vi "Acquire.vi"(3 "Correction and Conversion":dbl[](array[numeric]), 5 "Timing":T9={"Resolution (ms)"=0.0, "index"=0, "Duty cycle array size"=0, "Pre-scan rest (ms)"=2000}, 7 "Averaging and Conversion":T2, 9 "Method Output":T1, 11 "Data In":dbl[][](array[numeric]), 13 "Average In":dbl[][](array[numeric]), 16 "Calibration?":bool, 19 "Arduino In":cluster{"error in":errorcluster, "LINX  in":T3}) -> (2 "Stop condition":bool, 6 "Acquisition":T10, 10 "Data Out":dbl[][](array[numeric]), 12 "Average Out":dbl[][](array[numeric]), 14 "Arduino Out":cluster{"error out":errorcluster, "LINX out":T3})   [LabVIEW 2022 SP3]
uses:
  <vilib>/MakerHub/LINX/Private/Type Defs/LINX Ref.ctl
  <vilib>/MakerHub/LINX/Private/Type Defs/Platform.ctl
  <vilib>/MakerHub/LINX/Private/Type Defs/Interface.ctl
  <vilib>/MakerHub/LINX/Private/Device/Type Defs/LINX Device Config.ctl
  <vilib>/MakerHub/LINX/Private/Device/Type Defs/TCP Config.ctl
  <vilib>/MakerHub/LINX/Private/Device/Type Defs/Channels.ctl
  <vilib>/MakerHub/LINX/Public/Peripherals/PWM/PWM Set Duty Cycle 1 Chan.vi
  <vilib>/MakerHub/LINX/Public/Peripherals/Analog/Analog Read 1 Chan.vi
  <vilib>/Analysis/baseanly.llb/Mean (DBL).vi
  <vilib>/MakerHub/LINX/Public/Peripherals/Analog/Analog Read N Chans.vi
  <vilib>/MakerHub/LINX/Private/Local IO/LinxAnalogRead.vi
  <vilib>/MakerHub/LINX/Public/Utilities/Check Channel.vi
  <vilib>/MakerHub/LINX/Public/Peripherals/PWM/PWM Set Duty Cycle N Chans.vi
  <vilib>/MakerHub/LINX/Private/Utilties/Generate Error.vi
  <vilib>/MakerHub/LINX/LMH-LINX.lvlib
  <vilib>/Analysis/NI_AALBase.lvlib
  <vilib>/MakerHub/LINX/Private/Device/Device.lvlib
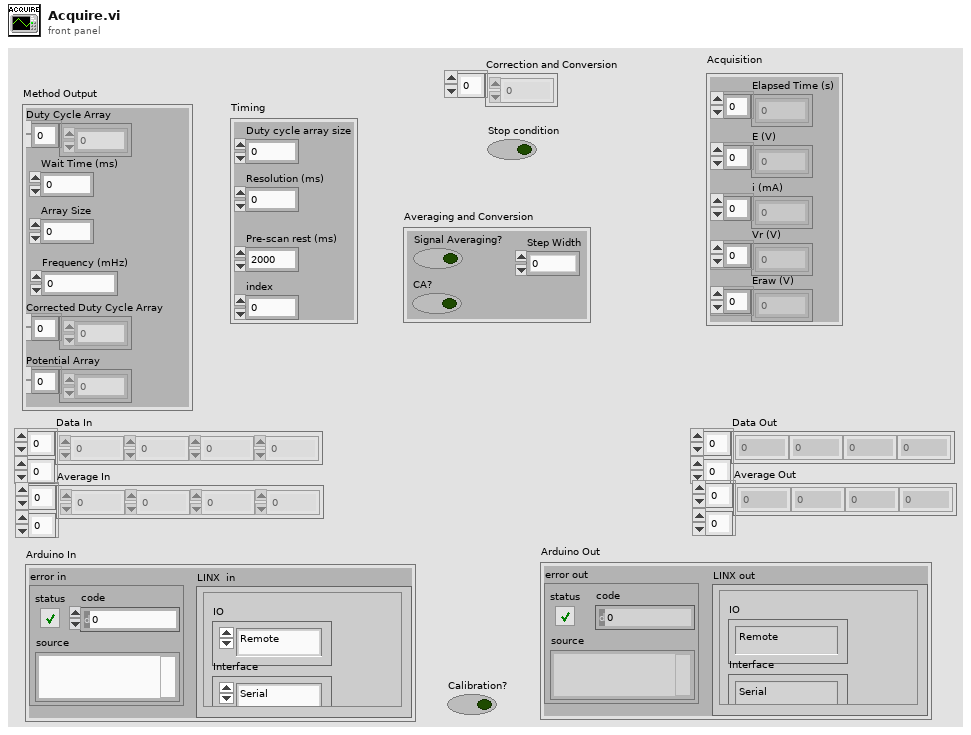
[diagram p1: front panel]
types:
  T1 = cluster{"Duty Cycle Array":dbl[], "Wait Time (ms)":dbl, "Array Size":i32, "Frequency (mHz)":dbl, "Corrected Duty Cycle Array":dbl[], "Potential Array":dbl[]}
  T2 = cluster{"Signal Averaging?":bool, "CA?":bool, "Step Width":dbl}
  T3 = typedef "LMH-LINX.lvlib/LINX Ref.ctl" = cluster{"IO":T4, "Interface":T5, "LINX Device Config":T6}
  T4 = typedef "LMH-LINX.lvlib/Platform.ctl" = enum16{"Remote", "Local"}
  T5 = typedef "LMH-LINX.lvlib/Interface.ctl" = enum16{"Serial", "TCP"}
  T6 = typedef "LMH-LINX.lvlib/Device.lvlib/LINX Device Config.ctl" = cluster{"Interface":T5, "COM Port":refnum<visa-resource-name>, "TCP Configuration":T7, "Device Family":u8, "Device ID":u8, "Device Name":string, "TCP Ref":refnum<k5>, "Channels":T8}
  T7 = typedef "LMH-LINX.lvlib/Device.lvlib/TCP Config.ctl" = cluster{"IP Address":string, "Port":u16}
  T8 = typedef "LMH-LINX.lvlib/Channels.ctl" = cluster{"DI":u8[], "DO":u8[], "AI":u8[], "AO":u8[], "PWM":u8[], "QE":u8[], "UART":u8[], "I2C 2":u8[], "SPI":u8[], "CAN":u8[], "Servo":u8[], "AI Ref (V)":dbl, "AI Resolution (Bits)":u8, "AO Ref (V)":dbl, "AO Resolution (Bits)":u8}
  T9 = cluster{"Resolution (ms)":dbl, "index":i32, "Duty cycle array size":i32, "Pre-scan rest (ms)":u32}
  T10 = cluster{"Elapsed Time (s)":dbl[], "E (V)":dbl[], "i (mA)":dbl[], "Vr (V)":dbl[], "Eraw (V)":dbl[]}
  T11 = cluster{"Error Out":errorcluster, "LINX Resource":T3}
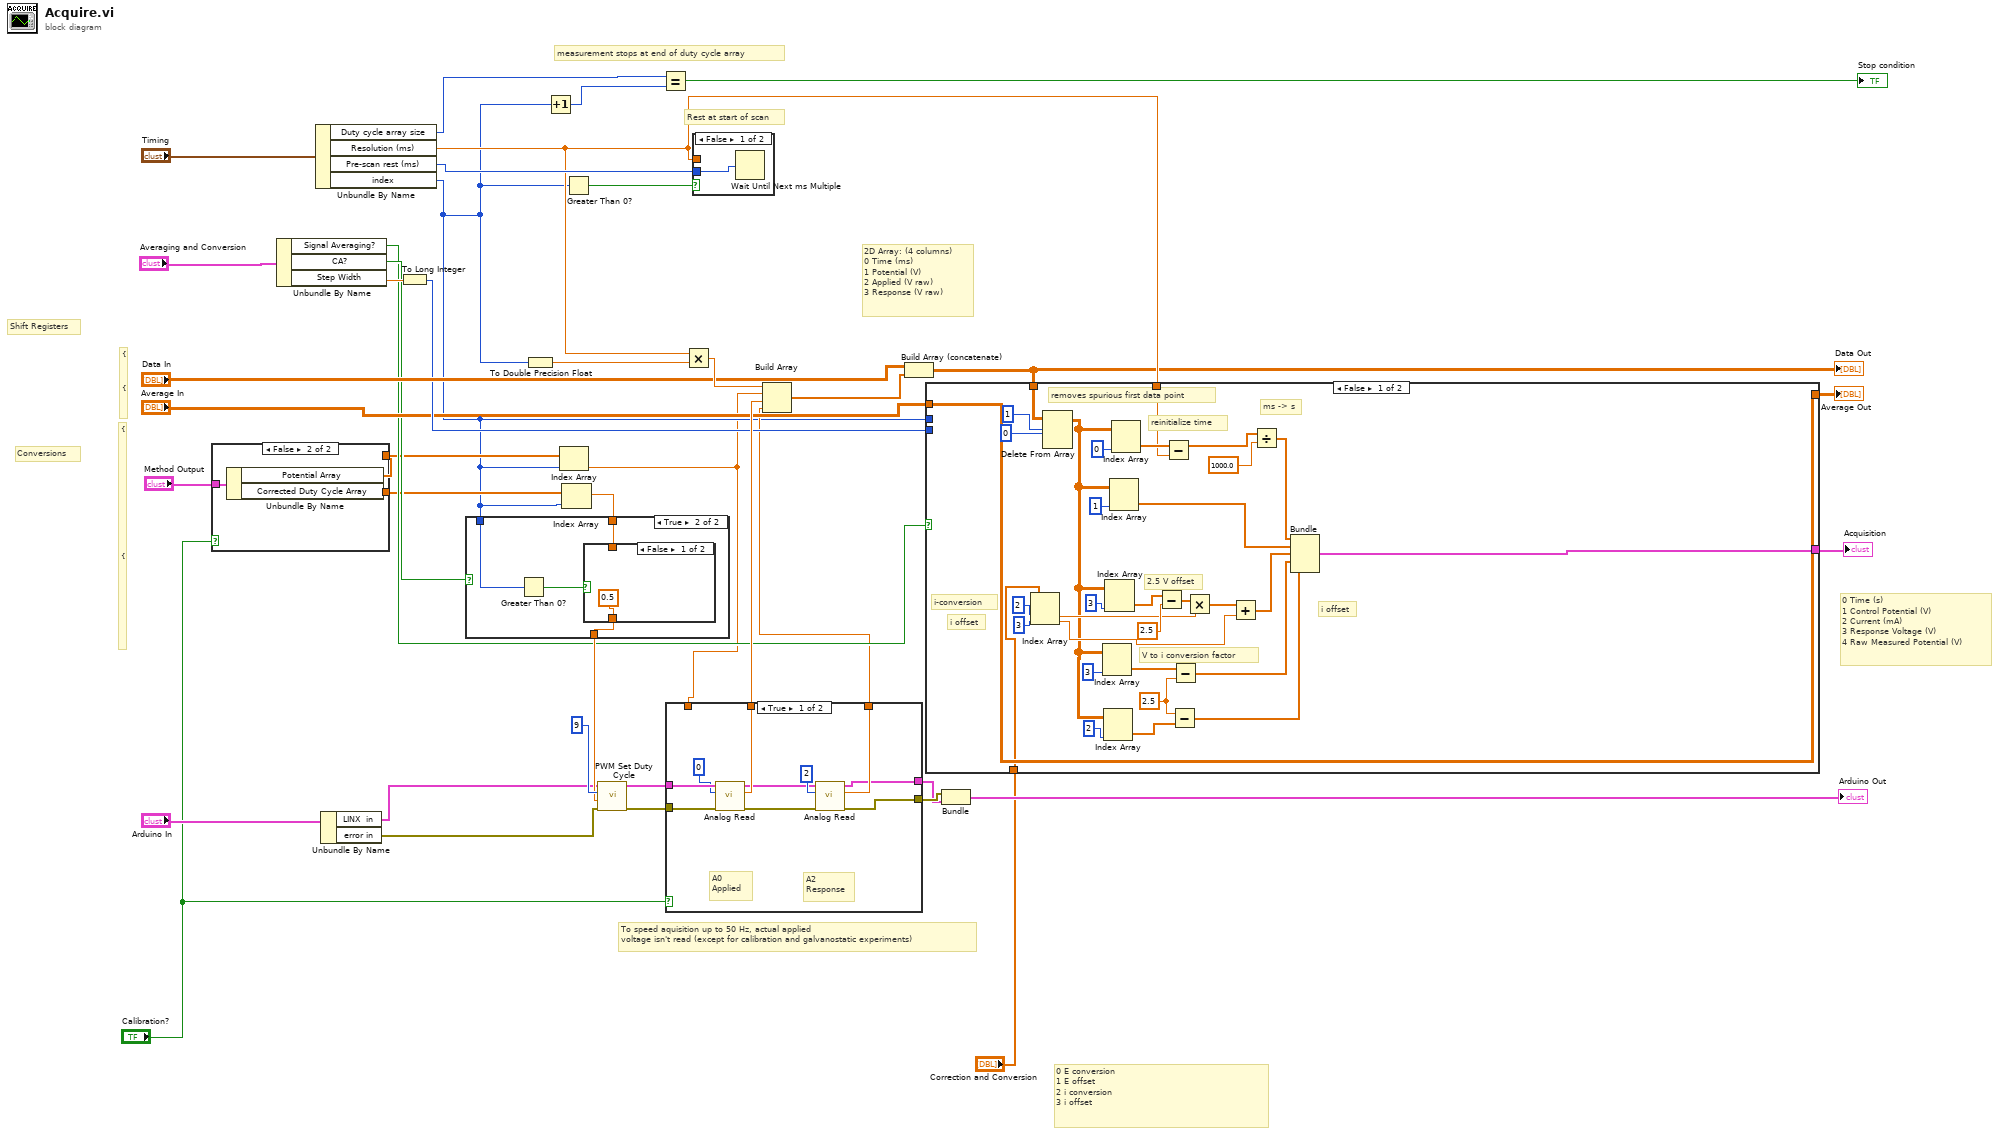
[diagram p0: block diagram]
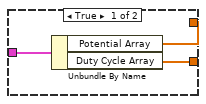
[diagram p2: hidden frame]
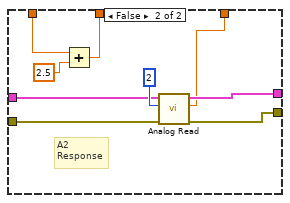
[diagram p3: hidden frame]
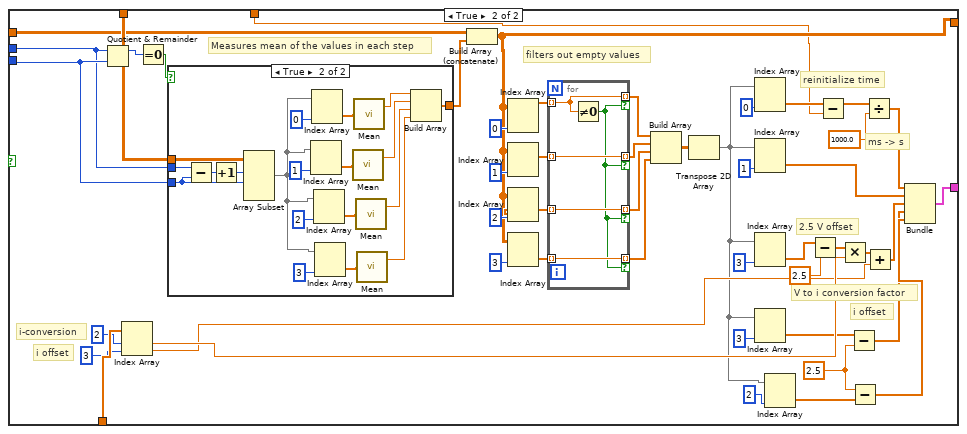
[diagram p4: hidden frame]
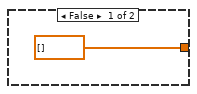
[diagram p5: hidden frame]
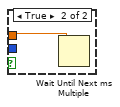
[diagram p8: hidden frame]
diagram:
  # "0 E conversion\n1 E offset\n2 i conversion \n3 i offset"
  # "0 Time (s)\n1 Control Potential (V)\n2 Current (mA)\n3 Response Voltage (V)\n4 Raw Measured Potential (V)"
  # "To speed aquisition up to 50 Hz, actual applied\nvoltage isn't read (except for calibration and galvanostatic experiments)"
  # "Shift Registers"
  # "{\n\n\n\n{"
  # "2D Array: (4 columns)\n0 Time (ms)\n1 Potential (V)\n2 Applied (V raw)\n3 Response (V raw)"
  # "Conversions"
  # "{\n\n\n\n\n\n\n\n\n\n\n\n\n\n\n{"
  # "Rest at start of scan"
  # "measurement stops at end of duty cycle array"
  n1 = case shown="False" "Calibration?" {
    tunnel: "Method Output" -> [w43 w46]
    tunnel: [w42 w45] -> w7
    tunnel: [w41 w44] -> w6
    frame True {
      n2 = Unbundle By Name(w43) -> ("Potential Array"=w41:dbl[], "Duty Cycle Array"=w42:dbl[])
    }
    frame False {
      n3 = Unbundle By Name(w46) -> ("Potential Array"=w44:dbl[], "Corrected Duty Cycle Array"=w45:dbl[])
    }
  }
  n4 = Unbundle By Name("Averaging and Conversion") -> ("Signal Averaging?"=w13:bool, "CA?"=w14:bool, "Step Width"=w15:dbl)
  n5 = Unbundle By Name("Timing") -> ("Duty cycle array size"=w28:i32, "Resolution (ms)"=w22:dbl, "Pre-scan rest (ms)"=w27:u32, "index"=w5:i32)
  n6 = Unbundle By Name("Arduino In") -> ("LINX  in"=w25:T3, "error in"=w24:errorcluster)
  n7 = To Long Integer(number=w15) -> (32bit integer=w20:i32)
  n8 = To Double Precision Float(number=w5) -> (double precision float=w12:dbl)
  n9 = Increment(x=w5) -> (x+1=w35:i32)
  n10 = Index Array(array=w6, index=w5) -> (element=w4:dbl)
  n11 = Index Array(array=w7, index=w5) -> (element=w30:dbl)
  n12 = case shown="True" w14 {
    tunnel: w5 -> [_ w51]
    tunnel: [w47 w49] -> w31
    tunnel: w30 -> [w47 w48]
    frame False {
    }
    frame True {
      n13 = Greater Than 0?(x=w51) -> (x > 0?=w50:bool)
      n14 = case shown="False" w50 {
        tunnel: [0.5 w53] -> w49
        tunnel: w48 -> [_ w53]
        frame False {
        }
        frame True {
        }
      }
    }
  }
  n15 = Greater Than 0?(x=w5) -> (x > 0?=w36:bool)
  n16 = call-poly <vilib>:"PWM Set Duty Cycle.vi"("Error In"=w24, "Duty Cycle (0-1)"=w31, "PWM Channel"=u8 9 ("DO Channel"), "LINX Resource"=w25) -> ("Error Out"=w39:errorcluster, "LINX Resource"=w38:T3)  [unwired: 6 in]
  n17 = Equal?(x=w28, y=w35) -> (x = y?=→"Stop condition":bool)
  n18 = case shown="True" "Calibration?" {
    tunnel: w39 -> [w63 w69]
    tunnel: w38 -> [w62 w68]
    tunnel: [w60 w65] -> w33
    tunnel: w4 -> [_ w66]
    tunnel: [w56 w70] -> w11
    tunnel: [w55 w67] -> w10
    tunnel: [w54 w71] -> w9
    frame True {
      # "A2\nResponse"
      # "A0\nApplied"
      n19 = call-poly <vilib>:"Analog Read.vi"("Error In"=w63, "Analog Channel"=u8 0, "LINX Resource"=w62) -> ("Error Out"=w59:errorcluster, "Voltage"=w60:dbl, "LINX Resource"=w57:T3)  [unwired: 5 in, 1 out]
      n20 = call-poly <vilib>:"Analog Read.vi"("Error In"=w59, "Analog Channel"=u8 2, "LINX Resource"=w57) -> ("Error Out"=w56:errorcluster, "Voltage"=w55:dbl, "LINX Resource"=w54:T3)  [unwired: 5 in, 1 out]
    }
    frame False {
      # "A2\nResponse"
      n21 = Add(x=w66, y=2.5) -> (x+y=w65:dbl)
      n22 = call-poly <vilib>:"Analog Read.vi"("Error In"=w69, "Analog Channel"=u8 2, "LINX Resource"=w68) -> ("Error Out"=w70:errorcluster, "Voltage"=w67:dbl, "LINX Resource"=w71:T3)  [unwired: 5 in, 1 out]
    }
  }
  n23 = Multiply(x=w22, y=w12) -> (x*y=w34:dbl)
  n24 = case shown="False" w36 {
    tunnel: w22 -> [_ w74]
    tunnel: w27 -> [w73 _]
    frame False {
      n25 = Wait Until Next ms Multiple(millisecond multiple=w73) -> ()  [unwired: 1 out]
    }
    frame True {
      n26 = Wait Until Next ms Multiple(millisecond multiple=w74) -> ()  [unwired: 1 out]
    }
  }
  n27 = Build Array(w34, w4, w33, w10) -> (w32:dbl[])
  n28 = Build Array (concatenate)("Data In", w32) -> (w17:dbl[][])
  "Data Out" <- w17
  n29 = case shown="False" w13 {
    tunnel: [w94 w107] -> w1
    tunnel: w22 -> [w92 w124]
    tunnel: w17 -> [w91 w151]
    tunnel: w20 -> [_ w153]
    tunnel: w5 -> [_ w152]
    tunnel: [w90 w136] -> w18
    tunnel: "Average In" -> [w90 w149]
    tunnel: "Correction and Conversion" -> [w82 w119]
    frame False {
      w75 = 2.5
      # "i offset"
      # "i-conversion"
      # "i offset"
      # "reinitialize time"
      # "V to i conversion factor"
      # "2.5 V offset"
      # "ms -> s"
      # "removes spurious first data point"
      n30 = Index Array(array=w82, index #1=2 ("index"), index #2=3 ("index")) -> (element #1=w84:dbl, element #2=w83:dbl)
      n31 = Delete From Array(array=w91, length=1, index (row)=0) -> (array with subset deleted=w81:dbl[][])  [unwired: 1 in, 1 out]
      n32 = Index Array(array=w81, index (col)=3 ("disabled index (col)")) -> (element=w76:dbl[])  [unwired: 1 in]
      n33 = Index Array(array=w81, index (col)=2 ("disabled index (col)")) -> (element=w79:dbl[])  [unwired: 1 in]
      n34 = Index Array(array=w81, index (col)=3 ("disabled index (col)")) -> (element=w99:dbl[])  [unwired: 1 in]
      n35 = Index Array(array=w81, index (col)=1 ("disabled index (col)")) -> (element=w95:dbl[])  [unwired: 1 in]
      n36 = Index Array(array=w81, index (col)=0 ("disabled index (col)")) -> (element=w103:dbl[])  [unwired: 1 in]
      n37 = Subtract(x=w99, y=2.5) -> (x-y=w97:dbl[])
      n38 = Subtract(x=w103, y=w92) -> (x-y=w93:dbl[])
      n39 = Subtract(x=w75, y=w79) -> (x-y=w78:dbl[])
      n40 = Subtract(x=w76, y=w75) -> (x-y=w77:dbl[])
      n41 = Multiply(x=w97, y=w84) -> (x*y=w88:dbl[])
      n42 = Add(x=w88, y=w83) -> (x+y=w87:dbl[])
      n43 = Divide(x=w93, y=1000.0) -> (x/y=w96:dbl[])
      n44 = Bundle(w96, w95, w87, w77, w78) -> (w94:cluster{dbl[], dbl[], dbl[], dbl[], dbl[]})  [unwired: 1 in]
    }
    frame True {
      w108 = 2.5
      # "i offset"
      # "i offset"
      # "i-conversion"
      # "reinitialize time"
      # "V to i conversion factor"
      # "2.5 V offset"
      # "ms -> s"
      # "filters out empty values"
      # "Measures mean of the values in each step"
      n45 = Quotient & Remainder(x=w152, y=w153) -> (x-y*floor(x/y)=w155:i32)  [unwired: 1 out]
      n46 = Index Array(array=w119, index #1=2 ("index"), index #2=3 ("index")) -> (element #1=w116:dbl, element #2=w115:dbl)
      n47 = Equal To 0?(x=w155) -> (x = 0?=w154:bool)
      n48 = case shown="True" w154 {
        tunnel: w151 -> [_ w180]
        tunnel: w153 -> [_ w163]
        tunnel: [dbl[] [] w179] -> w150
        tunnel: w152 -> [_ w164]
        frame False {
        }
        frame True {
          n49 = Subtract(x=w164, y=w163) -> (x-y=w165:i32)
          n50 = Increment(x=w165) -> (x+1=w162:i32)
          n51 = Array Subset(array=w180, index (row)=w162, length (row)=w163) -> (w169:dbl[][])  [unwired: 2 in]
          n52 = Index Array(array=w169, index (col)=1 ("disabled index (col)")) -> (element=w175:dbl[])  [unwired: 1 in]
          n53 = Index Array(array=w169, index (col)=0 ("disabled index (col)")) -> (element=w177:dbl[])  [unwired: 1 in]
          n54 = Index Array(array=w169, index (col)=2 ("disabled index (col)")) -> (element=w172:dbl[])  [unwired: 1 in]
          n55 = Index Array(array=w169, index (col)=3 ("disabled index (col)")) -> (element=w171:dbl[])  [unwired: 1 in]
          n56 = call-poly <vilib>:"Mean.vi"("X"=w175) -> ("mean"=w168:dbl)  [unwired: 1 out]
          n57 = call-poly <vilib>:"Mean.vi"("X"=w177) -> ("mean"=w176:dbl)  [unwired: 1 out]
          n58 = call-poly <vilib>:"Mean.vi"("X"=w172) -> ("mean"=w167:dbl)  [unwired: 1 out]
          n59 = call-poly <vilib>:"Mean.vi"("X"=w171) -> ("mean"=w166:dbl)  [unwired: 1 out]
          n60 = Build Array(w176, w168, w167, w166) -> (w179:dbl[])
        }
      }
      n61 = Build Array (concatenate)(w149, w150) -> (w136:dbl[][])
      n62 = Index Array(array=w136, index (col)=0 ("disabled index (col)")) -> (element=w141:dbl[])  [unwired: 1 in]
      n63 = Index Array(array=w136, index (col)=1 ("disabled index (col)")) -> (element=w142:dbl[])  [unwired: 1 in]
      n64 = Index Array(array=w136, index (col)=2 ("disabled index (col)")) -> (element=w143:dbl[])  [unwired: 1 in]
      n65 = Index Array(array=w136, index (col)=3 ("disabled index (col)")) -> (element=w144:dbl[])  [unwired: 1 in]
      n66 = for {
        tunnel: [w160] -> w145 mode=indexing if=w156
        tunnel: w141 -> [w160] mode=indexing
        tunnel: w142 -> [w159] mode=indexing
        tunnel: w143 -> [w158] mode=indexing
        tunnel: w144 -> [w157] mode=indexing
        tunnel: [w159] -> w146 mode=indexing if=w156
        tunnel: [w158] -> w147 mode=indexing if=w156
        tunnel: [w157] -> w148 mode=indexing if=w156
        n67 = Not Equal To 0?(x=w160) -> (x != 0?=w156:bool)
      }
      n68 = Build Array(w145, w146, w147, w148) -> (w123:dbl[][])
      n69 = Transpose 2D Array(2D array=w123) -> (transposed array=w112:dbl[][])
      n70 = Index Array(array=w112, index (col)=0 ("disabled index (col)")) -> (element=w135:dbl[])  [unwired: 1 in]
      n71 = Index Array(array=w112, index (col)=1 ("disabled index (col)")) -> (element=w131:dbl[])  [unwired: 1 in]
      n72 = Index Array(array=w112, index (col)=3 ("disabled index (col)")) -> (element=w134:dbl[])  [unwired: 1 in]
      n73 = Index Array(array=w112, index (col)=3 ("disabled index (col)")) -> (element=w110:dbl[])  [unwired: 1 in]
      n74 = Index Array(array=w112, index (col)=2 ("disabled index (col)")) -> (element=w113:dbl[])  [unwired: 1 in]
      n75 = Subtract(x=w134, y=2.5) -> (x-y=w133:dbl[])
      n76 = Subtract(x=w135, y=w124) -> (x-y=w130:dbl[])
      n77 = Multiply(x=w133, y=w116) -> (x*y=w120:dbl[])
      n78 = Subtract(x=w110, y=w108) -> (x-y=w109:dbl[])
      n79 = Subtract(x=w108, y=w113) -> (x-y=w111:dbl[])
      n80 = Divide(x=w130, y=1000.0) -> (x/y=w132:dbl[])
      n81 = Add(x=w120, y=w115) -> (x+y=w121:dbl[])
      n82 = Bundle(w132, w131, w121, w109, w111) -> (w107:cluster{dbl[], dbl[], dbl[], dbl[], dbl[]})  [unwired: 1 in]
    }
  }
  "Acquisition" <- w1
  "Average Out" <- w18
  n83 = Bundle("Error Out"=w11, "LINX Resource"=w9) -> (→"Arduino Out":T11)  [unwired: 1 in]
